vi "Get Timer From XML.vi"(11 "body":string) -> (0 "error out":errorcluster, 3 "Cluster":T1)   [LabVIEW 2013]
uses:
  Timer_Details_Ctrl.ctl
  <vilib>/xml/Close Reference(Node).vi
  <vilib>/xml/NI_XML.lvlib
  <resource>/objmgr/DOMUserDefRef.rc
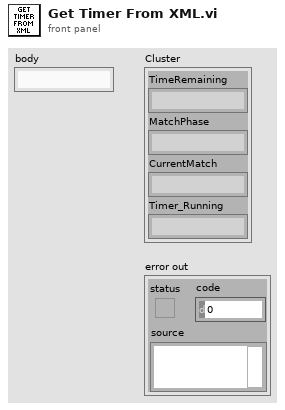
[diagram p1: front panel]
types:
  T1 = typedef "Timer_Details_Ctrl.ctl" = cluster{"TimeRemaining":string, "MatchPhase":string, "CurrentMatch":string, "Timer_Running":string}
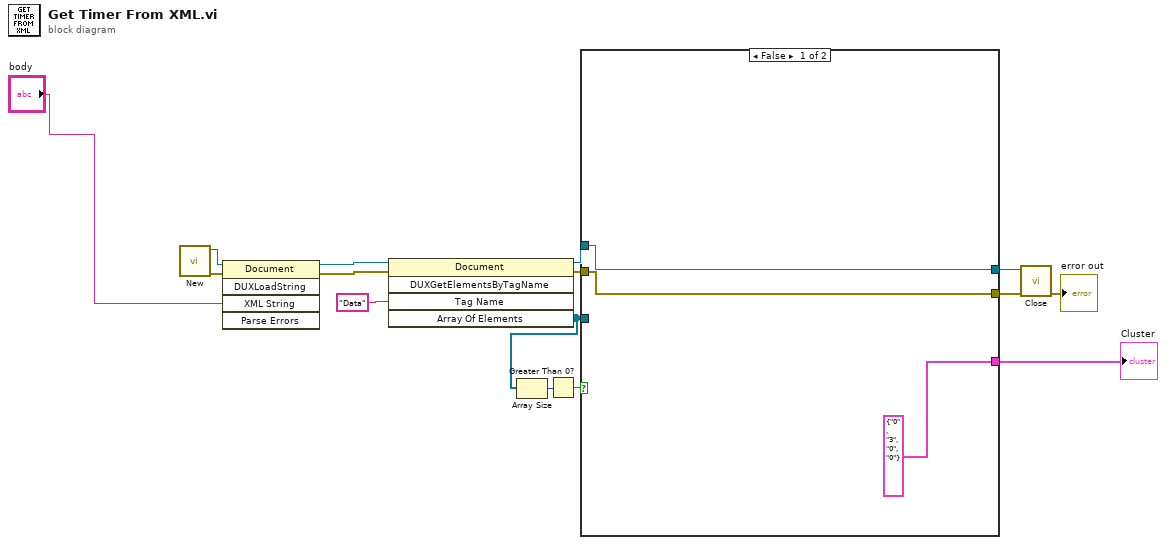
[diagram p0: block diagram]
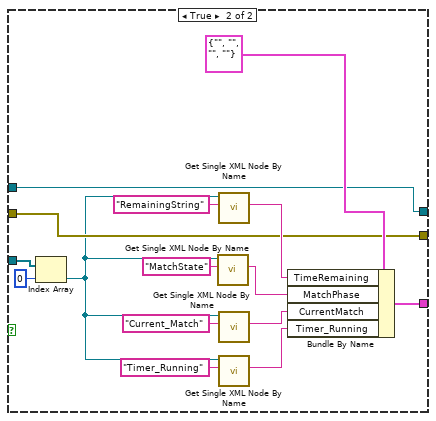
[diagram p2: hidden frame]
diagram:
  n1 = call <vilib>:"New.vi"() -> ("error out"=w7:errorcluster, "DOM document out"=w4:refnum<k20>)  [unwired: 8 in]
  n2 = invoke class="Document" method="DUXLoadString"(reference=w4, error in=w7, "XML String"="body") -> (reference out=w5:refnum<k20>, error out=w6:errorcluster)  [unwired: 2 in, 3 out]
  n3 = invoke class="Document" method="DUXGetElementsByTagName"(reference=w5, error in=w6, "Tag Name"="Data") -> (reference out=w12:refnum<k20>, error out=w14:errorcluster, "Array Of Elements"=w10:refnum<k20>[])  [unwired: 2 in, 2 out]
  n4 = Array Size(array=w10) -> (size(s)=w8:i32)
  n5 = Greater Than 0?(x=w8) -> (x > 0?=w9:bool)
  n6 = case shown="False" w9 {
    tunnel: [T1 {"TimeRemaining"="0", "MatchPhase"="3", "CurrentMatch"="0", "Timer_Running"="0"} w32] -> w2
    tunnel: w10 -> [_ w31]
    tunnel: [w18 w21] -> w11
    tunnel: w12 -> [w18 w21]
    tunnel: [w17 w20] -> w13
    tunnel: w14 -> [w17 w20]
    frame False {
    }
    frame True {
      n7 = Index Array(array=w31, index=0) -> (element=w19:refnum<k20>)
      n8 = call "Get Single XML Node By Name.vi"("Tag Name"="MatchState", "Parent Element"=w19) -> ("node text"=w24:string)  [unwired: 7 in, 2 out]
      n9 = call "Get Single XML Node By Name.vi"("Tag Name"="RemainingString", "Parent Element"=w19) -> ("node text"=w25:string)  [unwired: 7 in, 2 out]
      n10 = call "Get Single XML Node By Name.vi"("Tag Name"="Current_Match", "Parent Element"=w19) -> ("node text"=w23:string)  [unwired: 7 in, 2 out]
      n11 = call "Get Single XML Node By Name.vi"("Tag Name"="Timer_Running", "Parent Element"=w19) -> ("node text"=w22:string)  [unwired: 7 in, 2 out]
      n12 = Bundle By Name(cluster=T1 {"TimeRemaining"="", "MatchPhase"="", "CurrentMatch"="", "Timer_Running"=""}, "TimeRemaining"=w25, "MatchPhase"=w24, "CurrentMatch"=w23, "Timer_Running"=w22) -> (w32:T1)
    }
  }
  "Cluster" <- w2
  n13 = call-poly <vilib>:"Close.vi"("error in (no error)"=w13, "node"=w11) -> ("error out"=→"error out":errorcluster)  [unwired: 7 in]
